vi "Helper - System Time.vi"(7 "Date&Time":T1(ring), 8 "Error In":errorcluster) -> (0 "Error Out":errorcluster, 1 "Date & Time":string, 2 "Time":string, 3 "Date":string, 5 "Date & Time (WinFileFormat)":string)   [LabVIEW 2014, in "EventLogger_Actor.lvlib"]
uses:
  EventLogger_Actor.lvlib
panel:
  # "Connector Pane"
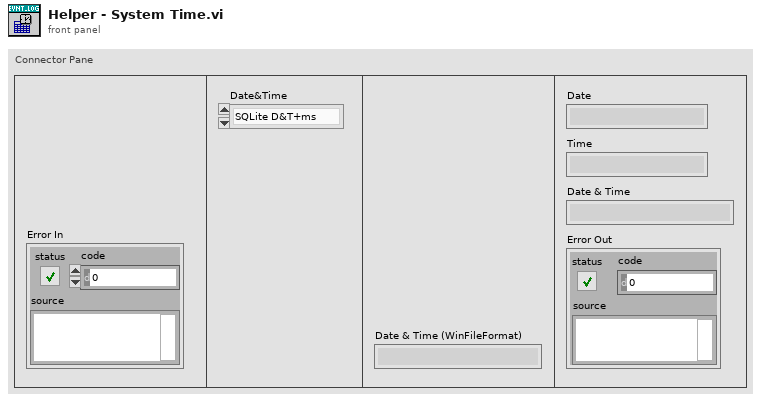
[diagram p1: front panel]
types:
  T1 = enum16{"SQLite D&T+ms", "SQLite D&T", "Gen D&T+ms", "Gen D&T"}
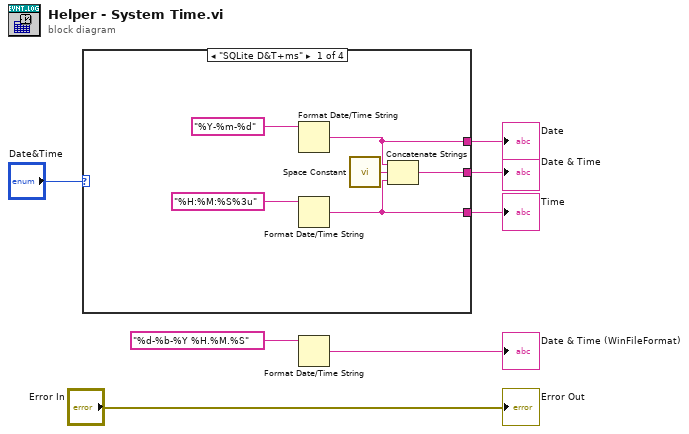
[diagram p0: block diagram]
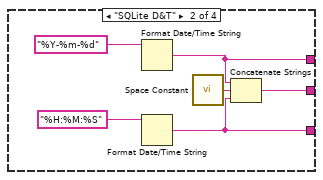
[diagram p2: hidden frame]
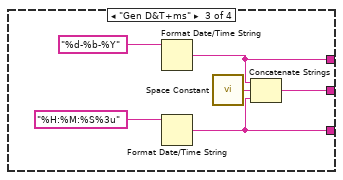
[diagram p3: hidden frame]
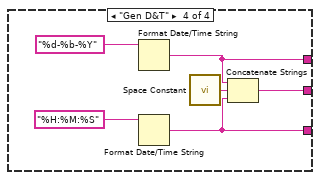
[diagram p4: hidden frame]
diagram:
  n1 = case shown="\"SQLite D&T+ms\"" "Date&Time" {
    tunnel: [w10 w16 w22 w28] -> w2
    tunnel: [w9 w14 w21 w26] -> w1
    tunnel: [w8 w15 w20 w27] -> w3
    frame "SQLite D&T+ms" {
      n2 = Format Date/Time String(time format string (%c)="%Y-%m-%d") -> (date/time string=w8:string)  [unwired: 2 in]
      n3 = Format Date/Time String(time format string (%c)="%H:%M:%S%3u") -> (date/time string=w9:string)  [unwired: 2 in]
      n4 = call <vilib>:"Space Constant.vi"() -> ("String"=w13:string)
      n5 = Concatenate Strings(w8, w13, w9) -> (w10:string)
    }
    frame "SQLite D&T" {
      n6 = Format Date/Time String(time format string (%c)="%Y-%m-%d") -> (date/time string=w15:string)  [unwired: 2 in]
      n7 = Format Date/Time String(time format string (%c)="%H:%M:%S") -> (date/time string=w14:string)  [unwired: 2 in]
      n8 = call <vilib>:"Space Constant.vi"() -> ("String"=w19:string)
      n9 = Concatenate Strings(w15, w19, w14) -> (w16:string)
    }
    frame "Gen D&T+ms" {
      n10 = Format Date/Time String(time format string (%c)="%d-%b-%Y") -> (date/time string=w20:string)  [unwired: 2 in]
      n11 = Format Date/Time String(time format string (%c)="%H:%M:%S%3u") -> (date/time string=w21:string)  [unwired: 2 in]
      n12 = call <vilib>:"Space Constant.vi"() -> ("String"=w25:string)
      n13 = Concatenate Strings(w20, w25, w21) -> (w22:string)
    }
    frame "Gen D&T" {
      n14 = Format Date/Time String(time format string (%c)="%d-%b-%Y") -> (date/time string=w27:string)  [unwired: 2 in]
      n15 = Format Date/Time String(time format string (%c)="%H:%M:%S") -> (date/time string=w26:string)  [unwired: 2 in]
      n16 = call <vilib>:"Space Constant.vi"() -> ("String"=w31:string)
      n17 = Concatenate Strings(w27, w31, w26) -> (w28:string)
    }
  }
  "Date" <- w3
  "Time" <- w1
  "Date & Time" <- w2
  n18 = Format Date/Time String(time format string (%c)="%d-%b-%Y %H.%M.%S") -> (date/time string=→"Date & Time (WinFileFormat)":string)  [unwired: 2 in]
  "Error Out" <- "Error In"
